vi "CRYGraph Table Window.vi"() -> ()   [LabVIEW 2013]
uses:
  Control/CRYTable Property.ctl
  <vilib>/Utility/miscctls.llb/LVRowAndColumnTypeDef.ctl
  Control/CRYFlag Cluster.ctl
  SubVI/CRYData View Global.vi
  SubVI/CRYMain Sub Window Global.vi
  CRYCurveLibrary/Global/CRYCurve Library Global.vi
panel:
  in  "LoadFinish":bool
  out "Find LDown":bool
  out "Find LUp":bool
  in  "Type RDown":enum16{"Curves", "Values", "Results", "WFM"}(ring)
  out "Index RDown":i32
  in  "Type LUp":enum16{"Curves", "Values", "Results", "WFM"}(ring)
  out "Index LUp":i32
  out "AscendSort":bool
  in  "OpenProperty":bool
  out "PropertyTab":string
  out "Event Name":string
  out "ReportDrop":bool
  out "Index":i32
  out "Index LDown":i32
  in  "Type":enum16{"Curves", "Values", "Results", "WFM"}(ring)
  out "Cell Position":T1
  out "Cell Position Down":T1
  out "TotalPlot":u32
  out "Graph Ref":refnum<vi>
  out "Test":string
  in  "Cursor":string[][](table)
  out "Cursor Ref":refnum<vi>
  out "Queue Name":string
  in  "StateOut":bool
  in  "CursorShow":bool
  out "Table Property":T2 {"Precision" items=["Digits of precision", "Significant digits"]}
  in  "Type LDown":enum16{"Curves", "Values", "Results", "WFM"}(ring)
  out "Graph Number":i32
  in  "LegendShow":bool
  in  "stop":bool
  out "Legend Ref":refnum<vi>
  in  "Legend":i32(listbox) caption="Multicolumn Listbox"
  in  "GraphType":string
  out "Title Name":string
  in  "Table":string[][](table)
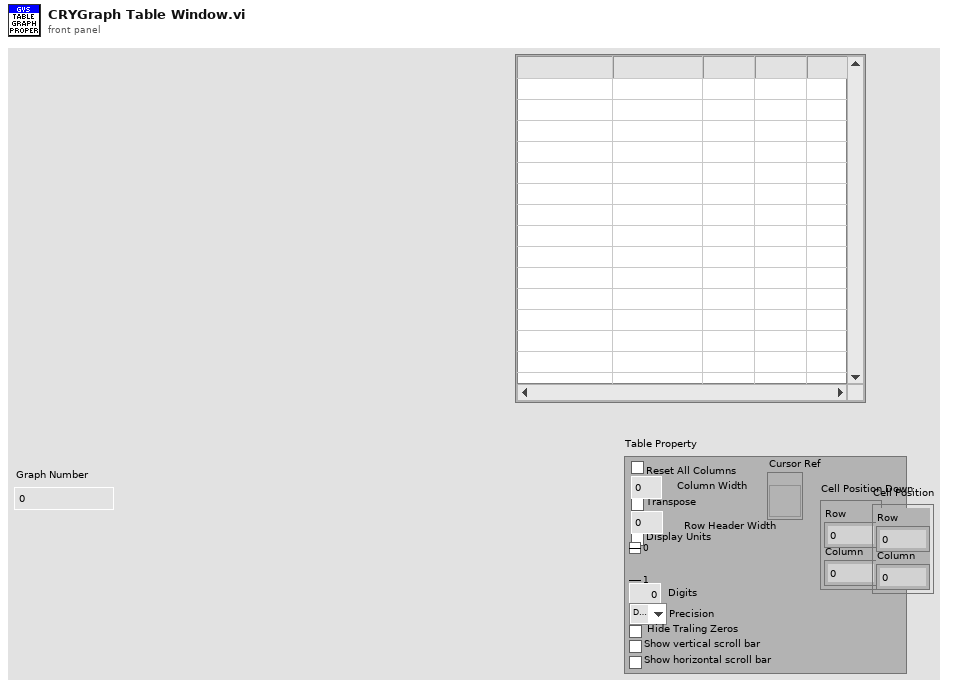
[diagram p1: front panel]
types:
  T1 = typedef "LVRowAndColumnTypeDef.ctl" = cluster{"Row":i32, "Column":i32}
  T2 = typedef "CRYTable Property.ctl" = cluster{"Reset All Columns":bool, "Transpose":bool, "Display Units":bool, "Notation":u16, "Digits":u16, "Precision":u16, "Hide Traling Zeros":bool, "Column Width":u16, "Row Header Width":u16, "Show vertical scroll bar":bool, "Show horizontal scroll bar":bool}
  T3 = typedef "CRYGraph Event.ctl" = cluster{"EvenName":string, "TitleName":string, "GraphName":string, "GraphType":string, "Data":variant, "Queue Name":string, "DataView Number":i32}
  T4 = typedef "CRYFlag Cluster.ctl" = cluster{"LegendShow":bool, "CellClick":bool, "Total Number":bool, "ScaleFitX":bool, "ScaleFitY":bool, "MapModeX":u8, "MapModeY":u8, "CursorShow":bool, "MagnitudeShow":bool, "PreviewShow":bool, "CursorEnabled":bool, "IntensityShow":bool, "PaletteShow":bool, "PhaseShow":bool, "XYShow":bool, "FrequencyShow":bool, "LegendVScrollShow":bool, "FrequencyVScrollShow":bool}
  T5 = enum16{"Curves", "Values", "Results", "WFM", "Others"}
  T6 = typedef "LVPoint32TypeDef.ctl" = cluster{"Horizontal":i32, "Vertical":i32}
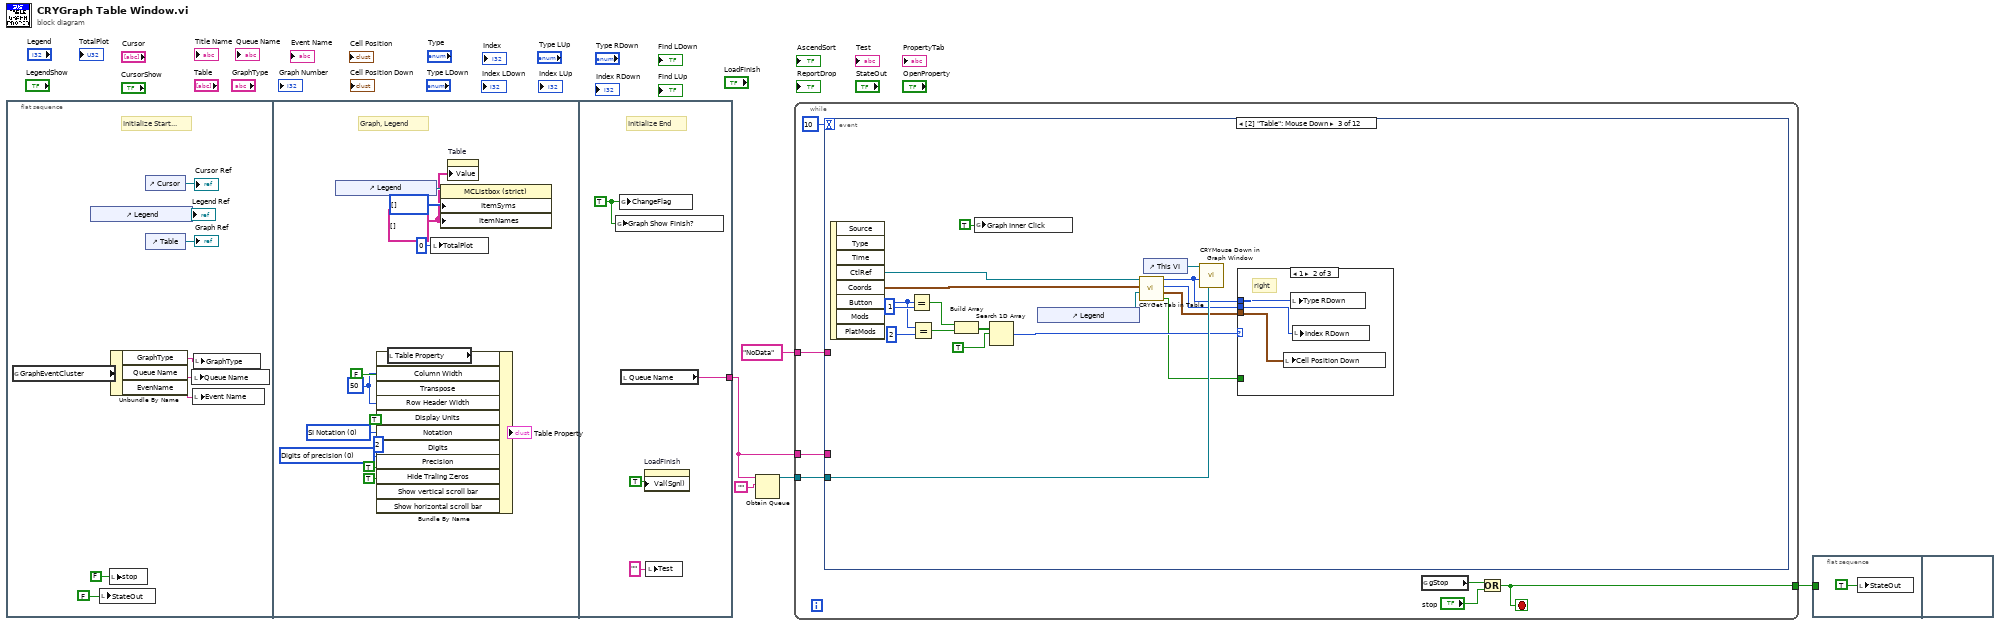
[diagram p0: block diagram]
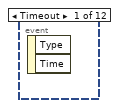
[diagram p2: hidden frame]
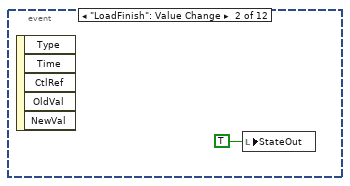
[diagram p3: hidden frame]
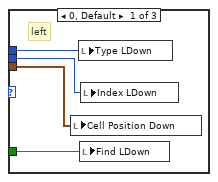
[diagram p4: hidden frame]
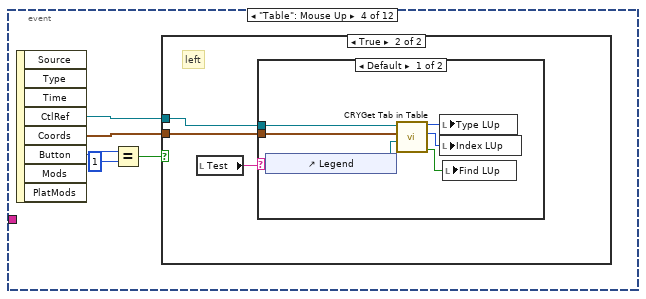
[diagram p6: hidden frame]
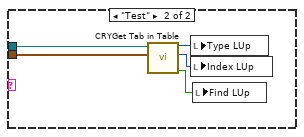
[diagram p8: hidden frame]
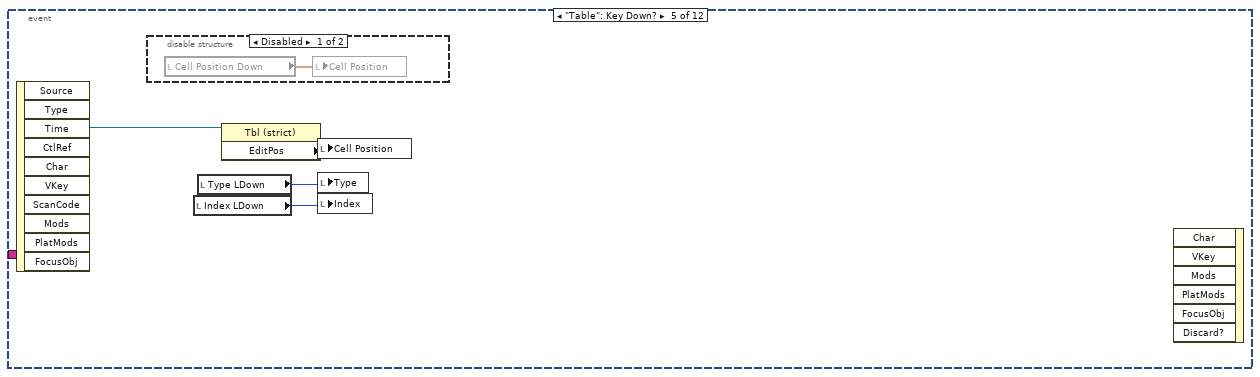
[diagram p9: hidden frame]
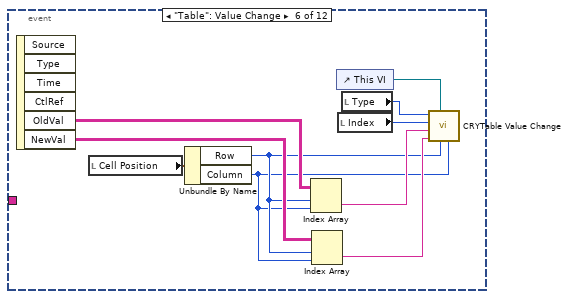
[diagram p11: hidden frame]
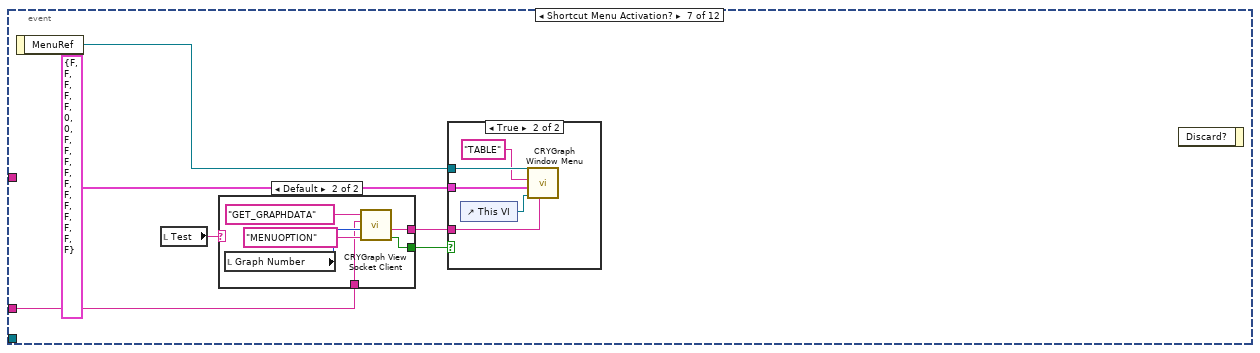
[diagram p12: hidden frame]
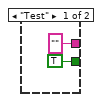
[diagram p13: hidden frame]
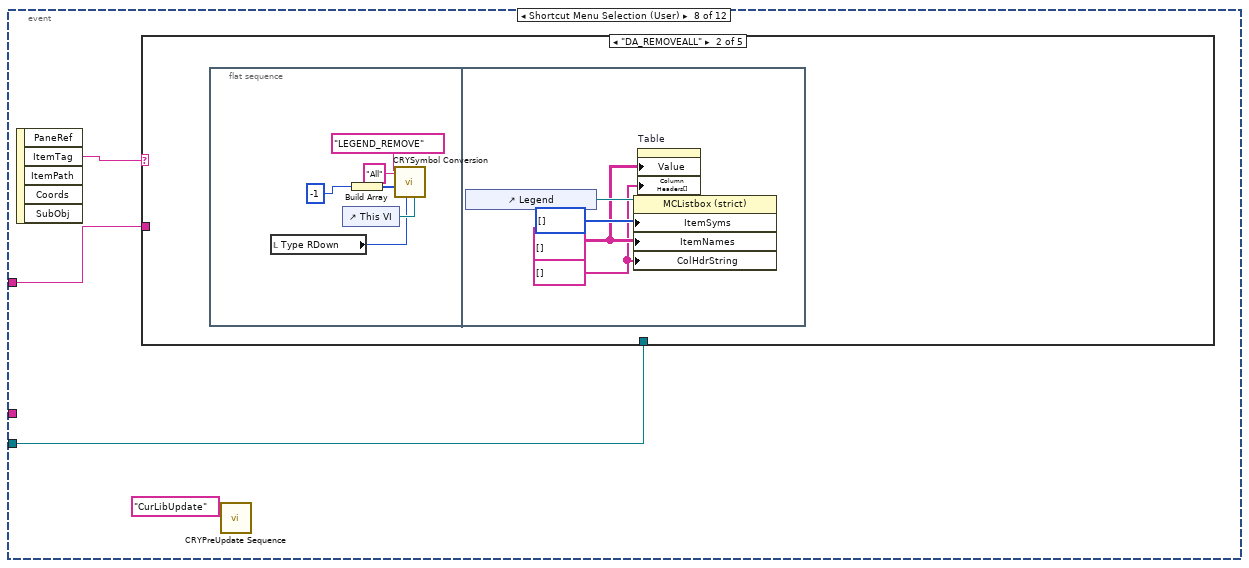
[diagram p15: hidden frame]
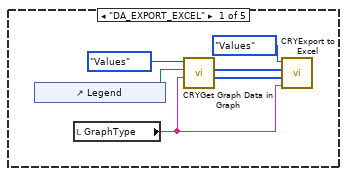
[diagram p16: hidden frame]
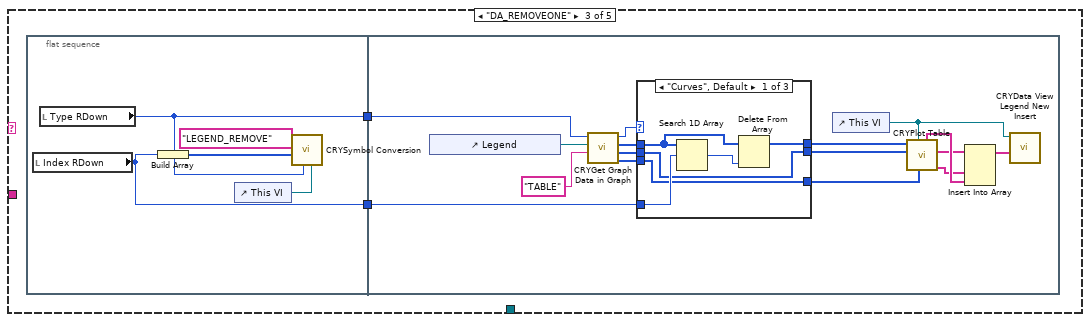
[diagram p17: hidden frame]
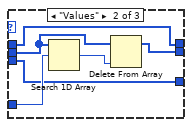
[diagram p18: hidden frame]
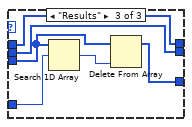
[diagram p19: hidden frame]
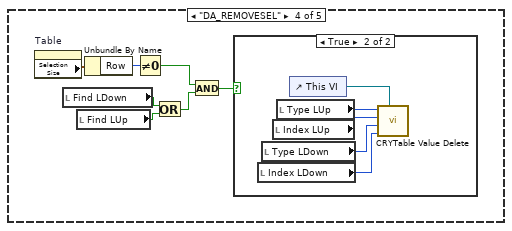
[diagram p20: hidden frame]
diagram:
  n1 = flat-sequence {
    tunnel: [w30] -> w1
    frame #0 {
      # "Initialize Start..."
      n2 = global read "CRYData View Global.vi" "GraphEventCluster"() -> (w7:T3)
      n3 = control-ref of="Legend"() -> (→"Legend Ref":refnum<vi>)
      n4 = local write "StateOut"(FALSE ("StateOut")) -> ()
      n5 = local write "stop"(FALSE ("stop")) -> ()
      n6 = Unbundle By Name(w7) -> ("GraphType"=w6:string, "Queue Name"=w8:string, "EvenName"=w9:string)
      n7 = control-ref of="Cursor"() -> (→"Cursor Ref":refnum<vi>)
      n8 = control-ref of="Table"() -> (→"Graph Ref":refnum<vi>)
      n9 = local write "Queue Name"(w8) -> ()
      n10 = local write "Event Name"(w9) -> ()
      n11 = local write "GraphType"(w6) -> ()
    }
    frame #1 {
      w15 = TRUE ("Show vertical scroll bar")
      w27 = u16 50 ("Column Width")
      w28 = FALSE ("Reset All Columns")
      w25 = u16 0 items=["Digits of precision", "Significant digits"] ("Precision")
      w23 = u16 0 items=["SI Notation", "Floating point"] ("Notation")
      w16 = string[][] [] ("Item Names")
      # "Graph, Legend"
      n12 = control-ref of="Legend"() -> (w18:refnum<vi>)
      n13 = local read "Table Property"() -> (w20:T2)
      n14 = Bundle By Name(cluster=w20, "Reset All Columns"=w28, "Column Width"=w27, "Transpose"=w28, "Row Header Width"=w27, "Display Units"=TRUE, "Notation"=w23, "Digits"=u16 2, "Precision"=w25, "Hide Traling Zeros"=TRUE, "Show vertical scroll bar"=w15, "Show horizontal scroll bar"=w15) -> (→"Table Property":T2)
      n15 = local write "TotalPlot"(u32 0 ("TotalPlot")) -> ()
      n16 = property on="Property Node" class="MCListbox (strict)"(reference=w18, "ItemSyms"=i32[] [] ("Item Symbols"), "ItemNames"=w16) -> ()  [unwired: 1 in, 2 out]
      n17 = property on="Table" class="Tbl (strict)"("Value"=w16) -> ()  [unwired: 2 in, 2 out]
    }
    frame #2 {
      w32 = TRUE ("ChangeFlag")
      # "Initialize End"
      n18 = global write "CRYData View Global.vi" "Graph Show Finish?"(w32) -> ()
      n19 = global write "CRYData View Global.vi" "ChangeFlag"(w32) -> ()
      n20 = local read "Queue Name"() -> (w30:string)
      n21 = property on="LoadFinish" class="Bool (strict)"("Val(Sgnl)"=TRUE ("Value (Signaling)")) -> ()  [unwired: 2 in, 2 out]
      n22 = local write "Test"("" ("Test")) -> ()
    }
  }
  n23 = Obtain Queue(name (unnamed)=w1, element data type="") -> (queue out=w4:refnum<queue>)  [unwired: 3 in, 2 out]
  n24 = while {
    tunnel: w4 -> [w39]
    tunnel: "NoData" ("input 2") -> [w36]
    tunnel: w1 -> [w34]
    tunnel: [w33] -> w2
    stop <- w33 stop-if-true
    n25 = event shown="[2] \"Table\": Mouse Down" {
      selector: _ -> [_ _ _ _ _ _ _ _ _ _ _ _]
      dyn-events: _ -> [_ _ _ _ _ _ _ _ _ _ _ _]
      timeout: 10 -> [_ _ _ _ _ _ _ _ _ _ _ _]
      tunnel: w39 -> [_ _ w57 _ _ _ _ w119 _ w235 w238 _]
      tunnel: w36 -> [_ _ _ _ _ _ _ w121 _ _ _ _]
      tunnel: w34 -> [_ _ _ _ _ _ w101 _ _ _ _ _]
      event Timeout {
        n26 = event-data() -> ()  [unwired: 3 out]
      }
      event "LoadFinish": Value Change {
        n27 = event-data() -> ()  [unwired: 6 out]
        n28 = local write "StateOut"(TRUE ("StateOut")) -> ()
      }
      event "Table": Mouse Down {
        n29 = event-data() -> ("CtlRef"=w56:refnum<vi>, "Coords"=w58:T6, "Button"=w53:u16)  [unwired: 6 out]
        n30 = Equal?(x=w53, y=u16 1) -> (x = y?=w52:bool)
        n31 = Equal?(x=w53, y=u16 2) -> (x = y?=w51:bool)
        n32 = Build Array(w52, w51) -> (w50:bool[])
        n33 = global write "CRYCurve Library Global.vi" "Graph Inner Click"(TRUE ("Graph Inner Click")) -> ()
        n34 = Search 1D Array(1D array=w50, element=TRUE) -> (index of element=w48:i32)  [unwired: 1 in]
        n35 = control-ref of="Legend"() -> (w46:refnum<vi>)
        n36 = call "CRYGet Tab in Table.vi"("Legend"=w46, "Mouse Point"=w58, "Table"=w56) -> ("bResult"=w42:bool, "Cell Position"=w43:T1, "Index"=w45:i32, "Type"=w44:enum16{"Curves", "Values", "Results", "WFM"})  [unwired: 5 out]
        n37 = control-ref of="This VI"() -> (w47:refnum<vi>)
        n38 = call "CRYMouse Down in Graph Window.vi"("Queue"=w57, "Selected Type"=w44, "pGraph VI In"=w47) -> ()  [unwired: 4 in, 5 out]
        n39 = case shown="1" w48 {
          tunnel: w44 -> [w62 w65 _]
          tunnel: w43 -> [w60 w64 _]
          tunnel: w45 -> [w61 w63 _]
          tunnel: w42 -> [w59 _ _]
          frame 0, Default {
            # "left"
            n40 = local write "Cell Position Down"(w60) -> ()
            n41 = local write "Type LDown"(w62) -> ()
            n42 = local write "Find LDown"(w59) -> ()
            n43 = local write "Index LDown"(w61) -> ()
          }
          frame 1 {
            # "right"
            n44 = local write "Cell Position Down"(w64) -> ()
            n45 = local write "Type RDown"(w65) -> ()
            n46 = local write "Index RDown"(w63) -> ()
          }
          frame -1 {
          }
        }
      }
      event "Table": Mouse Up {
        n47 = event-data() -> ("CtlRef"=w70:refnum<vi>, "Coords"=w69:T6, "Button"=w68:u16)  [unwired: 6 out]
        n48 = Equal?(x=w68, y=u16 1) -> (x = y?=w66:bool)
        n49 = case shown="True" w66 {
          tunnel: w70 -> [_ w73]
          tunnel: w69 -> [_ w72]
          frame False {
          }
          frame True {
            # "left"
            n50 = local read "Test"() -> (w71:string)
            n51 = case shown="Default" w71 {
              tunnel: w72 -> [w77 w82]
              tunnel: w73 -> [w79 w84]
              frame Default {
                n52 = control-ref of="Legend"() -> (w75:refnum<vi>)
                n53 = call "CRYGet Tab in Table.vi"("Legend"=w75, "Mouse Point"=w77, "Table"=w79) -> ("bResult"=w74:bool, "Index"=w76:i32, "Type"=w78:enum16{"Curves", "Values", "Results", "WFM"})  [unwired: 6 out]
                n54 = local write "Type LUp"(w78) -> ()
                n55 = local write "Index LUp"(w76) -> ()
                n56 = local write "Find LUp"(w74) -> ()
              }
              frame "Test" {
                n57 = call "CRYGet Tab in Table.vi"("Mouse Point"=w82, "Table"=w84) -> ("bResult"=w80:bool, "Index"=w81:i32, "Type"=w83:enum16{"Curves", "Values", "Results", "WFM"})  [unwired: 1 in, 6 out]
                n58 = local write "Type LUp"(w83) -> ()
                n59 = local write "Index LUp"(w81) -> ()
                n60 = local write "Find LUp"(w80) -> ()
              }
            }
          }
        }
      }
      event "Table": Key Down? {
        n61 = event-data() -> ("CtlRef"=w85:refnum<vi>)  [unwired: 10 out]
        n62 = disable-structure shown="Disabled" {
          frame Disabled {
            n63 = local read "Cell Position Down"() -> (w89:T1)
            n64 = local write "Cell Position"(w89) -> ()
          }
          frame Enabled {
          }
        }
        n65 = local read "Index LDown"() -> (w86:i32)
        n66 = local read "Type LDown"() -> (w87:enum16{"Curves", "Values", "Results", "WFM"})
        n67 = property class="Tbl (strict)"(reference=w85) -> ("EditPos"=w88:T1)  [unwired: 1 in, 2 out]
        n68 = local write "Cell Position"(w88) -> ()
        n69 = local write "Type"(w87) -> ()
        n70 = local write "Index"(w86) -> ()
        n71 = event-data() -> ()  [unwired: 7 in, 1 out]
      }
      event "Table": Value Change {
        n72 = event-data() -> ("OldVal"=w99:string[][], "NewVal"=w98:string[][])  [unwired: 5 out]
        n73 = local read "Cell Position"() -> (w90:T1)
        n74 = Unbundle By Name(w90) -> ("Row"=w93:i32, "Column"=w92:i32)
        n75 = Index Array(array=w99, index (row)=w93, index (col)=w92) -> (element=w95:string)
        n76 = Index Array(array=w98, index (row)=w93, index (col)=w92) -> (element=w94:string)
        n77 = control-ref of="This VI"() -> (w96:refnum<vi>)
        n78 = local read "Index"() -> (w91:i32)
        n79 = local read "Type"() -> (w97:enum16{"Curves", "Values", "Results", "WFM"})
        n80 = call "CRYTable Value Change.vi"("Column"=w92, "Row"=w93, "TableVI"=w96, "NewVal"=w94, "OldVal"=w95, "Index"=w91, "Type"=w97) -> ()  [unwired: 5 in]
      }
      event Shortcut Menu Activation? {
        n81 = event-data() -> ("MenuRef"=w102:refnum<k9>)  [unwired: 1 out]
        n82 = local read "Test"() -> (w100:string)
        n83 = case shown="Default" w100 {
          tunnel: ["" ("sData Out") w111] -> w105
          tunnel: [TRUE ("bResult Out") w110] -> w104
          tunnel: w101 -> [_ w108]
          frame "Test" {
          }
          frame Default {
            n84 = local read "Graph Number"() -> (w109:i32)
            n85 = call "CRYGraph View Socket Client.vi"("sOption"="MENUOPTION", "nData"=w109, "sData"=w108, "sAction"="GET_GRAPHDATA") -> ("bResult Out"=w110:bool, "sData Out"=w111:string)  [unwired: 4 in, 2 out]
          }
        }
        n86 = case shown="True" w104 {
          tunnel: w102 -> [_ w118]
          tunnel: T4 {"LegendShow"=FALSE, "CellClick"=FALSE, "Total Number"=FALSE, "ScaleFitX"=FALSE, "ScaleFitY"=FALSE, "MapModeX"=0, "MapModeY"=0, "CursorShow"=FALSE, "MagnitudeShow"=FALSE, "PreviewShow"=FALSE, "CursorEnabled"=FALSE, "IntensityShow"=FALSE, "PaletteShow"=FALSE, "PhaseShow"=FALSE, "XYShow"=FALSE, "FrequencyShow"=FALSE, "LegendVScrollShow"=FALSE, "FrequencyVScrollShow"=FALSE} ("Flag Cluster") -> [_ w116]
          tunnel: w105 -> [_ w115]
          frame False {
          }
          frame True {
            n87 = control-ref of="This VI"() -> (w114:refnum<vi>)
            n88 = call "CRYGraph Window Menu.vi"("MenuOption"=w115, "pGraph VI"=w114, "Flag Cluster"=w116, "Type"="TABLE", "Runtime Menu Ref In"=w118) -> ()  [unwired: 7 out]
          }
        }
        n89 = event-data() -> ()  [unwired: 1 in, 2 out]
      }
      event Shortcut Menu Selection (User) {
        n90 = event-data() -> ("ItemTag"=w122:string)  [unwired: 5 out]
        n91 = case shown="\"DA_REMOVEALL\"" w122 {
          selector: w122 -> [_ _ _ _ w194]
          tunnel: w121 -> [_ _ _ _ w193]
          tunnel: w119 -> [_ _ _ _ w192]
          frame "DA_EXPORT_EXCEL" {
            n92 = control-ref of="Legend"() -> (w123:refnum<vi>)
            n93 = local read "GraphType"() -> (w124:string)
            n94 = call "CRYGet Graph Data in Graph.vi"("Graph Type"=w124, "Legend Refnum"=w123, "Type In"=enum16{"Curves", "Values", "Results", "WFM"}."Values" ("Type")) -> ("Value Rows"=w125:i32[], "Rows"=w126:i32[])  [unwired: 1 in, 6 out]
            n95 = call "CRYExport to Excel.vi"("Graph Type"=w124, "Value  Rows"=w125, "Rows"=w126, "Type"=T5."Values") -> ()  [unwired: 8 out]
          }
          frame "DA_REMOVEALL" {
            n96 = flat-sequence {
              frame #0 {
                n97 = local read "Type RDown"() -> (w130:enum16{"Curves", "Values", "Results", "WFM"})
                n98 = control-ref of="This VI"() -> (w132:refnum<vi>)
                n99 = Build Array(-1 ("nData")) -> (w133:i32[])
                n100 = call "CRYSymbol Conversion.vi"("pGraph VI"=w132, "CurLib Tab Type"=w130, "nDatas"=w133, "sData"="All", "sActin"="LEGEND_REMOVE") -> ()  [unwired: 7 in]
              }
              frame #1 {
                w135 = string[] [] ("Column Header Strings[]")
                w136 = string[][] [] ("Item Names")
                n101 = control-ref of="Legend"() -> (w138:refnum<vi>)
                n102 = property on="Property Node" class="MCListbox (strict)"(reference=w138, "ItemSyms"=i32[] [] ("Item Symbols"), "ItemNames"=w136, "ColHdrString"=w135) -> ()  [unwired: 1 in, 2 out]
                n103 = property on="Table" class="Tbl (strict)"("Value"=w136, "Column Headers[]"=w135) -> ()  [unwired: 2 in, 2 out]
              }
            }
          }
          frame "DA_REMOVEONE" {
            n104 = flat-sequence {
              tunnel: [w144] -> w140
              tunnel: [w143] -> w139
              tunnel: w140 -> [w154]
              tunnel: w139 -> [w148]
              frame #0 {
                n105 = local read "Index RDown"() -> (w144:i32)
                n106 = local read "Type RDown"() -> (w143:enum16{"Curves", "Values", "Results", "WFM"})
                n107 = Build Array(w144) -> (w141:i32[])
                n108 = control-ref of="This VI"() -> (w142:refnum<vi>)
                n109 = call "CRYSymbol Conversion.vi"("pGraph VI"=w142, "CurLib Tab Type"=w143, "nDatas"=w141, "sActin"="LEGEND_REMOVE") -> ()  [unwired: 8 in]
              }
              frame #1 {
                n110 = control-ref of="Legend"() -> (w146:refnum<vi>)
                n111 = call "CRYGet Graph Data in Graph.vi"("Graph Type"="TABLE", "Legend Refnum"=w146, "Type In"=w148) -> ("Result Rows"=w151:i32[], "Value Rows"=w152:i32[], "Rows"=w155:i32[], "Type Out"=w161:enum16{"Curves", "Values", "Results", "WFM"})  [unwired: 1 in, 4 out]
                n112 = case shown="\"Curves\", Default" w161 {
                  tunnel: w155 -> [w166 w168 w175]
                  tunnel: w154 -> [w167 w173 w179]
                  tunnel: [w164 w168 w175] -> w153
                  tunnel: w152 -> [w163 w170 w174]
                  tunnel: w151 -> [w162 w171 w177]
                  tunnel: [w163 w169 w174] -> w150
                  tunnel: [w162 w171 w176] -> w149
                  frame "Curves", Default {
                    n113 = Search 1D Array(1D array=w166, element=w167) -> (index of element=w165:i32)  [unwired: 1 in]
                    n114 = Delete From Array(array=w166, index=w165) -> (array with subset deleted=w164:i32[])  [unwired: 1 in, 1 out]
                  }
                  frame "Values" {
                    n115 = Search 1D Array(1D array=w170, element=w173) -> (index of element=w172:i32)  [unwired: 1 in]
                    n116 = Delete From Array(array=w170, index=w172) -> (array with subset deleted=w169:i32[])  [unwired: 1 in, 1 out]
                  }
                  frame "Results" {
                    n117 = Search 1D Array(1D array=w177, element=w179) -> (index of element=w178:i32)  [unwired: 1 in]
                    n118 = Delete From Array(array=w177, index=w178) -> (array with subset deleted=w176:i32[])  [unwired: 1 in, 1 out]
                  }
                }
                n119 = control-ref of="This VI"() -> (w147:refnum<vi>)
                n120 = call "CRYPlot Table.vi"("Result Rows In"=w149, "pGraph VI In"=w147, "Value Rows In"=w150, "Curve Rows In"=w153) -> ("Value Name"=w157:string[], "Curve Name"=w156:string[], "Result Name"=w158:string[])  [unwired: 2 in, 3 out]
                n121 = Insert Into Array(array=w156, new element #1=w157, new element #2=w158) -> (w159:string[])  [unwired: 1 in]
                n122 = call "CRYData View Legend New Insert.vi"("ItemName Array"=w159, "pGraph VI In"=w147) -> ()  [unwired: 9 in, 1 out]
              }
            }
          }
          frame "DA_REMOVESEL" {
            n123 = property on="Table" class="Tbl (strict)"() -> ("Selection Size"=w186:T1)  [unwired: 2 in, 2 out]
            n124 = local read "Find LDown"() -> (w184:bool)
            n125 = local read "Find LUp"() -> (w183:bool)
            n126 = Unbundle By Name(w186) -> ("Row"=w185:i32)
            n127 = Not Equal To 0?(x=w185) -> (x != 0?=w182:bool)
            n128 = Or(x=w184, y=w183) -> (x .or. y?=w181:bool)
            n129 = And(x=w182, y=w181) -> (x .and. y?=w180:bool)
            n130 = case shown="True" w180 {
              frame False {
              }
              frame True {
                n131 = local read "Index LDown"() -> (w190:i32)
                n132 = local read "Type LDown"() -> (w187:enum16{"Curves", "Values", "Results", "WFM"})
                n133 = local read "Index LUp"() -> (w189:i32)
                n134 = local read "Type LUp"() -> (w188:enum16{"Curves", "Values", "Results", "WFM"})
                n135 = control-ref of="This VI"() -> (w191:refnum<vi>)
                n136 = call "CRYTable Value Delete.vi"("TableVI"=w191, "Index Down"=w190, "Type Down"=w187, "Index Up"=w189, "Type Up"=w188) -> ()  [unwired: 7 in]
              }
            }
          }
          frame Default {
            n137 = Search/Split String(string=w194, search string/char (-)="#") -> (substring before match=w199:string, match + rest of string=w196:string)  [unwired: 2 out]
            n138 = Decimal String To Number(string=w196, offset=1) -> (number=w198:i32)  [unwired: 2 out]
            n139 = case shown="0, Default" w198 {
              selector: w198 -> [_ w213]
              tunnel: w199 -> [w202 w215]
              tunnel: w193 -> [_ w212]
              tunnel: w192 -> [w206 w210]
              frame 0, Default {
                n140 = local read "GraphType"() -> (w200:string)
                n141 = local read "Graph Number"() -> (w207:i32)
                n142 = Equal?(x="DA_EXPORT_DOCUMENT" ("y"), y=w202) -> (x = y?=w205:bool)
                n143 = Select(t="ADD_DOC", s=w205, f=w202) -> (s? t:f=w201:string)
                n144 = Format Into String(w201, w200, w207, 0 ("input 3")) -> (resulting string=w208:string)  [unwired: 3 in, 1 out]
                n145 = Enqueue Element(queue=w206, element=w208) -> ()  [unwired: 1 in, 4 out]
              }
              frame 1..10 {
                n146 = flat-sequence {
                  tunnel: w215 -> [w218]
                  tunnel: [w218] -> w214
                  tunnel: w213 -> [w217]
                  tunnel: w212 -> [_]
                  tunnel: [w216] -> w211
                  tunnel: w214 -> [w222]
                  tunnel: w211 -> [w220]
                  tunnel: w210 -> [w219]
                  frame #0 {
                    n147 = call "CRYSet Graph Cluster Data.vi"("Graph Number"=w217) -> ("DataType"=w216:string)  [unwired: 2 in, 8 out]
                  }
                  frame #1 {
                    n148 = local read "Graph Number"() -> (w221:i32)
                    n149 = Format Into String(w222, w220, w221, 0 ("input 3")) -> (resulting string=w224:string)  [unwired: 3 in, 1 out]
                    n150 = Enqueue Element(queue=w219, element=w224) -> ()  [unwired: 1 in, 4 out]
                  }
                }
              }
            }
          }
        }
        n151 = call "CRYPreUpdate Sequence.vi"("EventName"="CurLibUpdate") -> ()  [unwired: 15 in]
      }
      event "Table": Drag Enter {
        n152 = event-data() -> ("Available Data Names"=w226:string[])  [unwired: 1 out]
        n153 = disable-structure shown="Disabled" {
          disable-tunnel: w226 -> [w229 _]
          disable-tunnel: [w227 TRUE] -> w225
          frame Disabled {
            n154 = Search 1D Array(1D array=w229, element="CRY_GRAPH_DATA") -> (index of element=w231:i32)  [unwired: 1 out]
            n155 = Not Equal?(x=w231, y=-1) -> (x != y?=w227:bool)
          }
          frame Enabled {
          }
        }
        n156 = event-data("Accepted?"=w225) -> ()  [unwired: 1 in, 1 out]
      }
      event "Table": Drop {
        n157 = event-data() -> ()  [unwired: 2 out]
        n158 = local read "Event Name"() -> (w233:string)
        n159 = control-ref of="This VI"() -> (w234:refnum<vi>)
        n160 = call "CRYDrop Data in Same Graph.vi"("pGraph VI"=w234, "Queue"=w235, "sAction"=w233) -> ("Accepted?"=w236:bool)  [unwired: 4 in, 4 out]
        n161 = event-data("Accepted?"=w236) -> ()  [unwired: 1 in, 1 out]
      }
      event "ReportDrop": Value Change {
        n162 = event-data() -> ()  [unwired: 7 out]
        n163 = local read "Event Name"() -> (w237:string)
        n164 = control-ref of="This VI"() -> (w239:refnum<vi>)
        n165 = call "CRYDrop Data in Same Graph.vi"("pGraph VI"=w239, "Queue"=w238, "sAction"=w237) -> ()  [unwired: 4 in, 5 out]
      }
      event "OpenProperty": Value Change {
        n166 = event-data() -> ()  [unwired: 7 out]
        n167 = flat-sequence {
          frame #0 {
            n168 = local read "PropertyTab"() -> (w240:string)
            n169 = control-ref of="This VI"() -> (w241:refnum<vi>)
            n170 = call "CRYGraph Property Window Main.vi"("TabName"=w240, "pGraph VI In"=w241) -> ()  [unwired: 1 in, 9 out]
          }
          frame #1 {
            n171 = local write "PropertyTab"("" ("PropertyTab")) -> ()
          }
        }
      }
    }
    n172 = global read "CRYMain Sub Window Global.vi" "gStop"() -> (w38:bool)
    n173 = Or(x=w38, y="stop") -> (x .or. y?=w33:bool)
  }
  n174 = flat-sequence {
    tunnel: w2 -> [_]
    frame #0 {
      n175 = local write "StateOut"(TRUE ("StateOut")) -> ()
    }
    frame #1 {
    }
  }
